vi "LUnit CLI Pre-Uninstall.vi"(10 "operations directory override":string, 11 "Variant":variant) -> (0 "error out":errorcluster, 3 "operation path":path)   [LabVIEW 2020]
doc: "VIPM pre-uninstall custom action for LUnit CLI.\n\nRemoves the LUnitCLI operation folder that LUnit CLI Post-Install.vi copied into the LabVIEW CLI Operations directory. The Operations directory is the first of these that exists:\n Windows: C:/Program Files (x86)/National Instruments/Shared/LabVIEW CLI/Operations/LUnitCLI\n Linux: /usr/local/natinst/nilvcli/Operations/LUnitCLI\n macOS: /Library/Application Support/National Instruments/LabVIEW CLI/Operations/LUnitCLI\nA folder that is not there is not an error. A folder that is there but cannot be deleted is reported in error out.\n\nThe override input exists for testing only. VIPM leaves it empty."
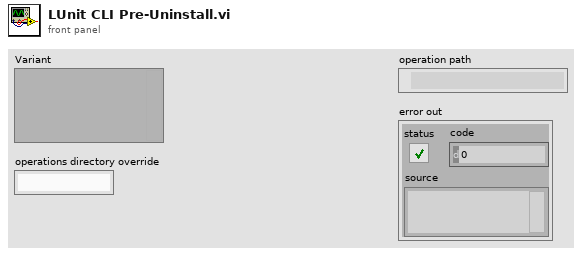
[diagram p1: front panel]
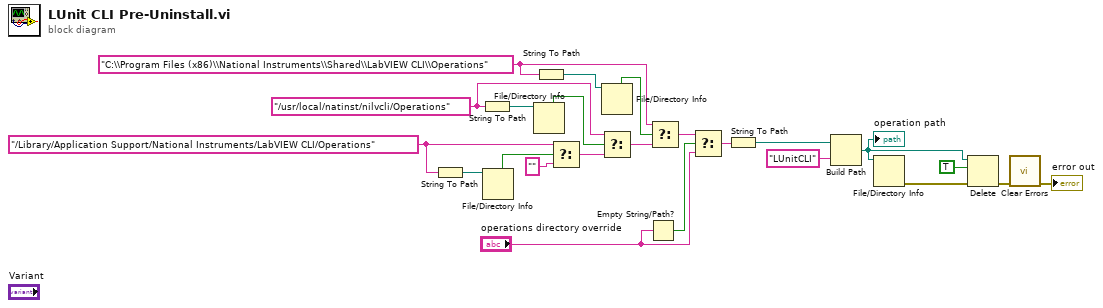
[diagram p0: block diagram]
diagram:
  w20 = "/Library/Application Support/National Instruments/LabVIEW CLI/Operations"
  w17 = "/usr/local/natinst/nilvcli/Operations"
  w14 = "C:\\Program Files (x86)\\National Instruments\\Shared\\LabVIEW CLI\\Operations"
  n1 = String To Path(string=w20) -> (path=w21:path)
  n2 = String To Path(string=w17) -> (path=w22:path)
  n3 = File/Directory Info(path=w21) -> (directory=w19:bool)  [unwired: 1 in, 6 out]
  n4 = File/Directory Info(path=w22) -> (directory=w16:bool)  [unwired: 1 in, 6 out]
  n5 = String To Path(string=w14) -> (path=w23:path)
  n6 = Select(t=w20, s=w19, f="") -> (s? t:f=w15:string)
  n7 = File/Directory Info(path=w23) -> (directory=w13:bool)  [unwired: 1 in, 6 out]
  n8 = Select(t=w17, s=w16, f=w15) -> (s? t:f=w12:string)
  n9 = Empty String/Path?(string/path="operations directory override") -> (empty?=w10:bool)
  n10 = Select(t=w14, s=w13, f=w12) -> (s? t:f=w11:string)
  n11 = Select(t=w11, s=w10, f="operations directory override") -> (s? t:f=w8:string)
  n12 = String To Path(string=w8) -> (path=w7:path)
  n13 = Build Path(base path=w7, name or relative path="LUnitCLI") -> (appended path=w3:path)
  "operation path" <- w3
  n14 = File/Directory Info(path=w3) -> (error out=w4:errorcluster)  [unwired: 1 in, 6 out]
  n15 = Delete(path (use dialog)=w3, entire hierarchy (F)=TRUE, error in=w4) -> (error out=w2:errorcluster)  [unwired: 2 in, 2 out]
  n16 = call <vilib>:"Clear Errors.vi"("error in (no error)"=w2) -> ("error out"=→"error out":errorcluster)  [unwired: 5 in, 1 out]
